vi "AxisResetError.vi"(8 "error in (no error)":errorcluster) -> (0 "error out":errorcluster)   [LabVIEW 2020, in "输出轴伺服.lvlib"]
uses:
  Servo_global.vi
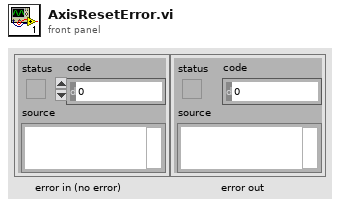
[diagram p1: front panel]
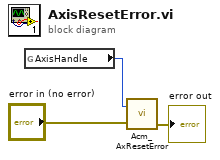
[diagram p0: block diagram]
diagram:
  n1 = global read "Servo_global.vi" "AxisHandle"() -> (w1:u32)
  n2 = call <userlib>:"Acm_AxResetError.vi"("Error Input(No Error)"="error in (no error)", "AxisHandle"=w1) -> ("Error Output"=→"error out":errorcluster)  [unwired: 2 out]
